vi "MGCC_DataLog_main.vi"   [LabVIEW 2016]
doc: "-----------------------------------------------------------------------------------------------------------------------\nCopyright <2019> <The University of Tennessee at Knoxville and the University of Tennessee Research Foundation>\nThis software is released under BSD-3 \nhttps://opensource.org/licenses/BSD-3-Clause \nAdditional license options available at https://utrf.tennessee.edu/industry/sample-agreements/\n-----------------------------------------------------------------------------------------------------------------------"
uses:
  Finite State Machine/Sub-VIs/MGCC_FntStaMach_gobal.vi
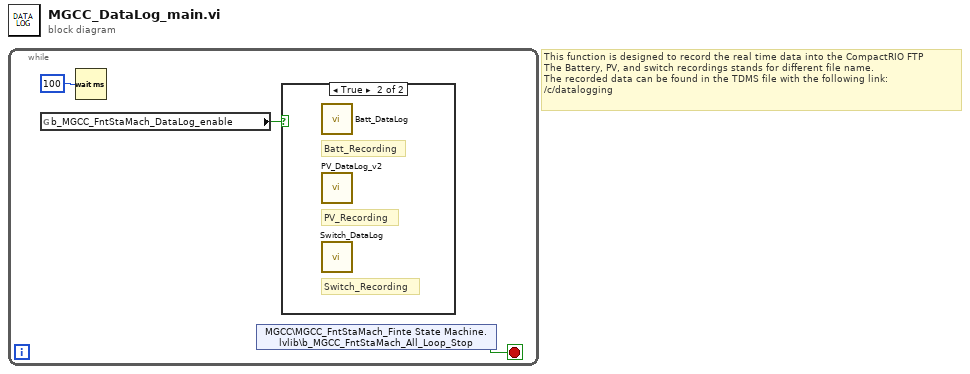
[diagram p0: block diagram]
diagram:
  # "This function is designed to record the real time data into the CompactRIO FTP\nThe Battery, PV, and switch recordings stands for different file name.\nThe recorded data can be found in the TDMS file with the following link:\n/c/datalogging"
  n1 = while {
    stop <- w2 stop-if-true
    n2 = global read "MGCC_FntStaMach_gobal.vi" "b_MGCC_FntStaMach_DataLog_enable"() -> (w1:bool)
    n3 = Wait (ms)(milliseconds to wait=u32 100) -> ()  [unwired: 1 out]
    n4 = shared-variable "MGCC\\MGCC_FntStaMach_Finte State Machine.lvlib\\b_MGCC_FntStaMach_All_Loop_Stop"() -> (w2:bool)  [unwired: 1 in, 1 out]
    n5 = case shown="True" w1 {
      frame False {
      }
      frame True {
        # "Switch_Recording"
        # "PV_Recording"
        # "Batt_Recording"
        n6 = call "Batt_DataLog.vi"() -> ()  [unwired: 1 in, 1 out]
        n7 = call "PV_DataLog_v2.vi"() -> ()  [unwired: 2 in]
        n8 = call "Switch_DataLog.vi"() -> ()  [unwired: 2 in]
      }
    }
  }
